vi "SRV_Parse Response (B).vi"(11 "#B Data in":string) -> (0 "number of bytes in buffer_data":i32, 1 "Beginning of buffer_data":string, 2 "remaining bytes in buffer_data":i32, 3 "#B Data dup":string, 4 "Got Beginning of Other Response?":bool, 5 "Read More?":bool, 6 "Beginning of Other Response":string)   [LabVIEW 2014]
panel:
  out "Command":string
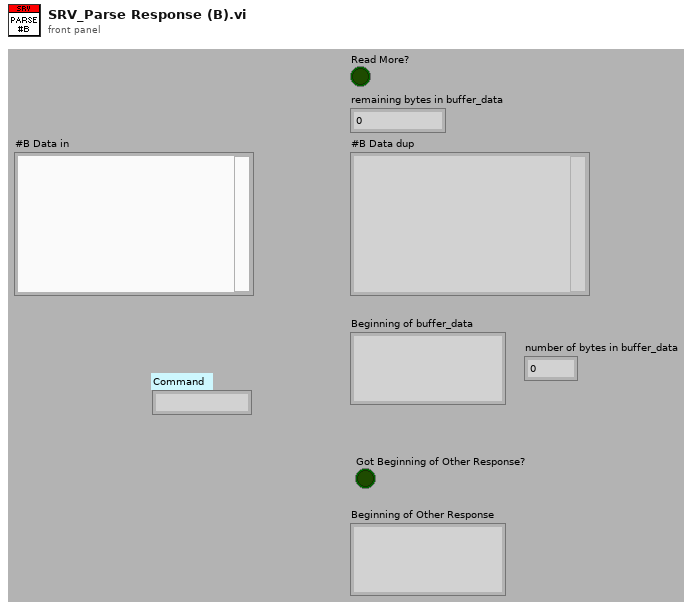
[diagram p1: front panel]
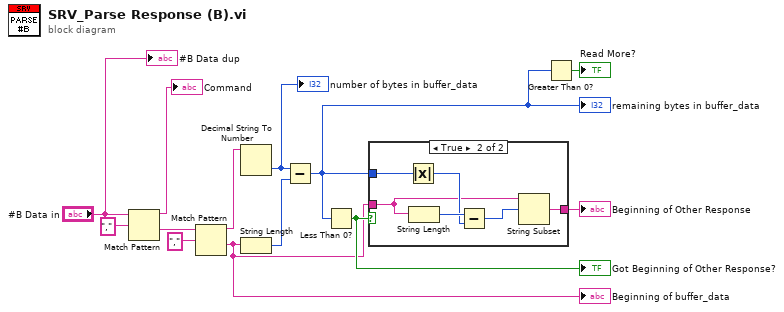
[diagram p0: block diagram]
diagram:
  n1 = Match Pattern(string="#B Data in", regular expression=",") -> (before substring=→"Command":string, after substring=w11:string)  [unwired: 1 in, 2 out]
  n2 = Match Pattern(string=w11, regular expression=",") -> (before substring=w9:string, after substring=w5:string)  [unwired: 1 in, 2 out]
  "Beginning of buffer_data" <- w5
  n3 = Decimal String To Number(string=w9) -> (number=w8:i32)  [unwired: 2 in, 1 out]
  "number of bytes in buffer_data" <- w8
  n4 = String Length(string=w5) -> (length=w7:i32)
  n5 = Subtract(x=w8, y=w7) -> (x-y=w3:i32)
  "remaining bytes in buffer_data" <- w3
  n6 = Less Than 0?(x=w3) -> (x < 0?=w6:bool)
  "Got Beginning of Other Response?" <- w6
  n7 = case shown="True" w6 {
    tunnel: w5 -> [_ w14]
    tunnel: w3 -> [_ w19]
    tunnel: [_ w15] -> w4
    frame False {
    }
    frame True {
      n8 = Absolute Value(x=w19) -> (abs(x)=w17:i32)
      n9 = String Length(string=w14) -> (length=w18:i32)
      n10 = Subtract(x=w18, y=w17) -> (x-y=w16:i32)
      n11 = String Subset(string=w14, offset (0)=w16) -> (substring=w15:string)  [unwired: 1 in]
    }
  }
  "Beginning of Other Response" <- w4
  n12 = Greater Than 0?(x=w3) -> (x > 0?=→"Read More?":bool)
  "#B Data dup" <- "#B Data in"
